vi "Enumerate video modes.vi"(1 "Video modes":u16(ring), 3 "Session In":T1="cam0") -> (0 "Error Out":errorcluster)   [LabVIEW 2014]
uses:
  <vilib>/userdefined/High Color/IMAQdx.ctl
  <vilib>/Utility/miscctls.llb/LVStringsAndValuesArrayTypeDef_U16.ctl
  <vilib>/vision/driver/IMAQdx.llb/IMAQdx Camera Control Mode.ctl
  <vilib>/vision/driver/NI_Vision_Acquisition_Software.lvlib
panel:
  # "PN 27/11/2014"
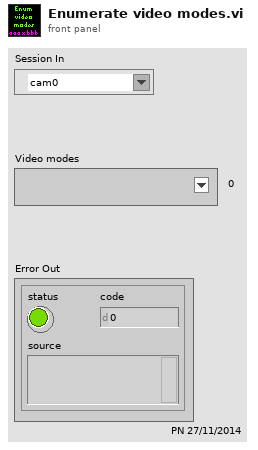
[diagram p1: front panel]
types:
  T1 = typedef "IMAQdx.ctl" = refnum<k21>
  T2 = typedef "NI_Vision_Acquisition_Software.lvlib/IMAQdx Camera Control Mode.ctl" = enum32{"Controller", "Listener"}
  T3 = typedef "LVStringsAndValuesArrayTypeDef_U16.ctl" = cluster{"String":string, "Value":u16}[]
  T4 = cluster{"Video Mode":u32, "Video Mode Name":string}[]
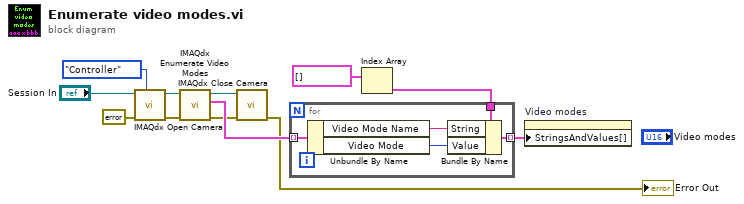
[diagram p0: block diagram]
diagram:
  n1 = call <vilib>:"IMAQdx Open Camera.vi"("Camera Control Mode"=IMAQdx_Camera_Control_Mode."Controller", "error in"=errorcluster {"status"=FALSE, "code"=0, "source"=""}, "Session In"="Session In") -> ("error out"=w5:errorcluster, "Session Out"=w6:T1)  [unwired: 7 in]
  n2 = call <vilib>:"IMAQdx Enumerate Video Modes.vi"("error in"=w5, "Session In"=w6) -> ("error out"=w4:errorcluster, "Video Modes"=w12:T4, "Session Out"=w3:T1)  [unwired: 6 in, 1 out]
  n3 = call <vilib>:"IMAQdx Close Camera.vi"("error in"=w4, "Session In"=w3) -> ("error out"=→"Error Out":errorcluster)  [unwired: 9 in]
  n4 = Index Array(array=T3 [] ("Strings And Values []")) -> (element=w10:cluster{"String":string, "Value":u16})  [unwired: 1 in]
  n5 = for {
    tunnel: w12 -> [w17] mode=indexing
    tunnel: w10 -> [w16]
    tunnel: [w13] -> w9 mode=indexing
    n6 = Unbundle By Name(w17) -> ("Video Mode Name"=w15:string, "Video Mode"=w14:u32)
    n7 = Bundle By Name(cluster=w16, "String"=w15, "Value"=w14) -> (w13:cluster{"String":string, "Value":u16})
  }
  n8 = property on="Video modes" class="Ring (strict)"("StringsAndValues[]"=w9) -> ()  [unwired: 2 in, 2 out]
